vi "Test0405.vi"() -> ()   [LabVIEW 2021]
panel:
  out "Waveform Graph":dbl[](graph)
  in  "stop":bool
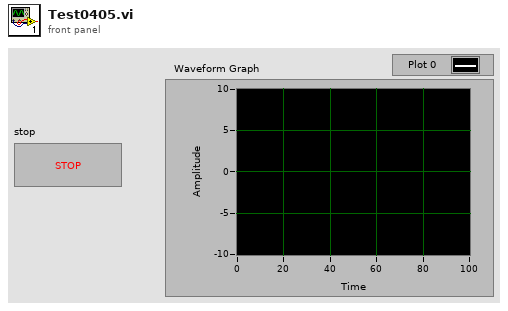
[diagram p1: front panel]
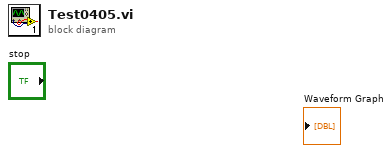
[diagram p0: block diagram]
diagram:
